vi "随机数发生器（高斯分布）.vi"(0 "标准差":dbl=1.0 format="%0.2f", 1 "种子":i32=-1, 2 "重置":bool) -> (4 "x1":dbl)   [LabVIEW 2012]
doc: "功能：\n\n产生高斯白噪声。\n\n基本算法：\n\nBox-Muller变换法。\n\ncsxcs_366创建"
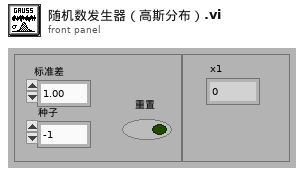
[diagram p1: front panel]
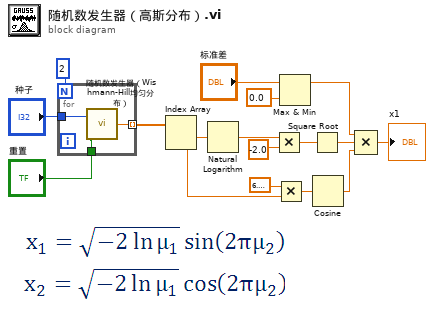
[diagram p0: block diagram]
diagram:
  n1 = for {
    N: 2 -> [_]
    tunnel: "种子" -> [w20]
    tunnel: [w19] -> w15 mode=indexing
    tunnel: "重置" -> [w18]
    n2 = call "随机数发生器（Wishmann-Hill均匀分布）.vi"("Seed"=w20, "Reset"=w18) -> ("Ui"=w19:dbl)  [unwired: 3 in]
  }
  n3 = Index Array(array=w15) -> (element #1=w14:dbl, element #2=w10:dbl)  [unwired: 2 in]
  n4 = Natural Logarithm(1:w14) -> (0:w13:dbl)
  n5 = Multiply(x=w13, y=-2.0) -> (x*y=w8:dbl)
  n6 = Multiply(x=6.283185307179586, y=w10) -> (x*y=w9:dbl)
  n7 = Max & Min(x="标准差", y=0.0) -> (max(x,y)=w2:dbl)  [unwired: 1 out]
  n8 = Square Root(x=w8) -> (sqrt(x)=w7:dbl)
  n9 = Cosine(x=w9) -> (cos(x)=w6:dbl)
  n10 = Compound Arithmetic op=MULTIPLY(w2, w7, w6) -> (→"x1":dbl)
